vi "Set Channel Names.vi"(10 "Data":dbl[](array[numeric]), 11 "file path (dialog if empty)":path) -> (2 "Channel Length":i32, 3 "new file path (Not A Path if cancelled)":path)   [LabVIEW 2019, in "Platform.lvlib" / "Platform.lvclass"]
uses:
  Platform.lvclass
  <vilib>/Utility/file.llb/Write Delimited Spreadsheet (string).vi
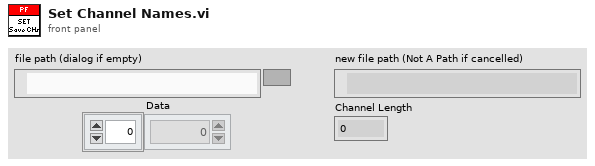
[diagram p1: front panel]
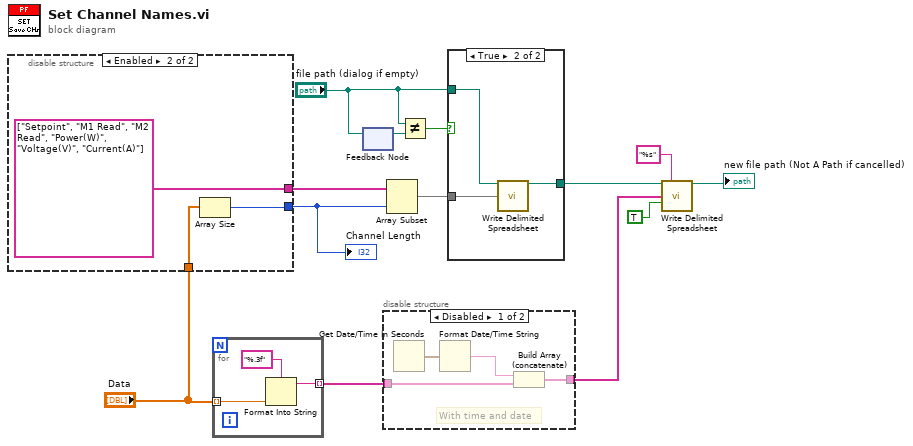
[diagram p0: block diagram]
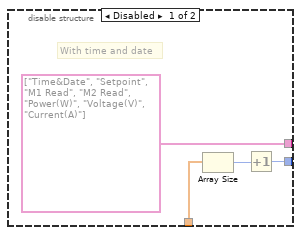
[diagram p3: hidden frame]
diagram:
  n1 = disable-structure shown="Enabled" {
    disable-tunnel: [string[] ["Time&Date", "Setpoint", "M1 Read", "M2 Read", "Power(W)", "Voltage(V)", "Current(A)"] string[] ["Setpoint", "M1 Read", "M2 Read", "Power(W)", "Voltage(V)", "Current(A)"]] -> w8
    disable-tunnel: "Data" -> [w16 w19]
    disable-tunnel: [w15 w18] -> w1
    frame Disabled {
      # "With time and date"
      n2 = Array Size(array=w16) -> (size(s)=w14:i32)
      n3 = Increment(x=w14) -> (x+1=w15:i32)
    }
    frame Enabled {
      n4 = Array Size(array=w19) -> (size(s)=w18:i32)
    }
  }
  "Channel Length" <- w1
  n5 = for {
    tunnel: "Data" -> [w23] mode=indexing
    tunnel: [w21] -> w4 mode=indexing
    n6 = Format Into String(format string="%.3f", w23) -> (resulting string=w21:string)  [unwired: 2 in, 1 out]
  }
  n7 = feedback #1() -> (w12:path)  [unwired: 1 in]
  n8 = feedback-in #1("file path (dialog if empty)") -> ()
  n9 = disable-structure shown="Disabled" {
    disable-tunnel: w4 -> [w26 w28]
    disable-tunnel: [w25 w28] -> w3
    frame Disabled {
      # "With time and date"
      n10 = Get Date/Time In Seconds() -> (seconds since 1Jan1904=w27:timestamp)
      n11 = Format Date/Time String(seconds (now)=w27) -> (date/time string=w24:string)  [unwired: 2 in]
      n12 = Build Array (concatenate)(w24, w26) -> (w25:string[])
    }
    frame Enabled {
    }
  }
  n13 = Array Subset(array=w8, length=w1) -> (w13:string[])  [unwired: 1 in]
  n14 = Not Equal?(x="file path (dialog if empty)", y=w12) -> (x != y?=w10:bool)
  n15 = case shown="True" w10 {
    tunnel: w13 -> [_ w32]
    tunnel: [w29 w31] -> w7
    tunnel: "file path (dialog if empty)" -> [w29 w30]
    frame False {
    }
    frame True {
      n16 = call-poly <vilib>:"Write Delimited Spreadsheet.vi"("file path (dialog if empty)"=w30, "1D data"=w32) -> ("new file path (Not A Path if cancelled)"=w31:path)  [unwired: 12 in, 1 out]
    }
  }
  n17 = call-poly <vilib>:"Write Delimited Spreadsheet.vi"("file path (dialog if empty)"=w7, "format (%s)"="%s" ("format (%.3f)"), "1D data"=w3, "append to file? (new file:F)"=TRUE) -> ("new file path (Not A Path if cancelled)"=→"new file path (Not A Path if cancelled)":path)  [unwired: 10 in, 1 out]
